vi "check if settings file exists.vi"(8 "error in (no error)":errorcluster, 11 "Autofocus in":refnum<class "Autofocus.lvclass">) -> (0 "error out":errorcluster, 2 "settings file exists?":bool, 3 "Autofocus out":refnum<class "Autofocus.lvclass">)   [LabVIEW 2012, in "Autofocus.lvclass"]
uses:
  Autofocus.lvclass
  <vilib>/Distrio/Murmex/Murmex/Murmex.lvclass
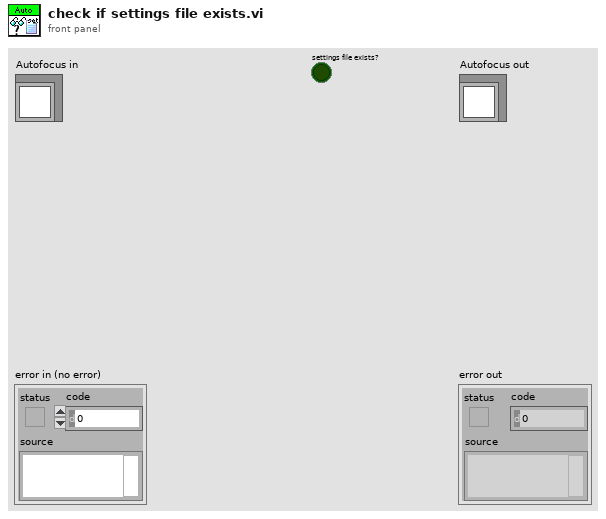
[diagram p1: front panel]
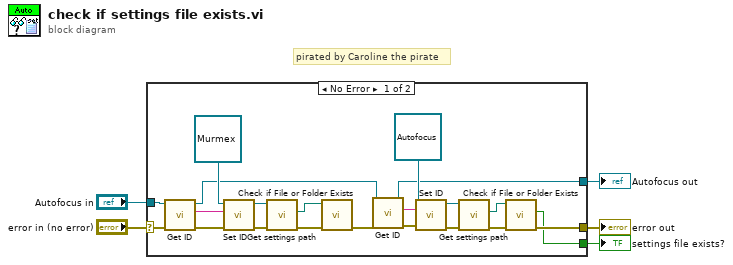
[diagram p0: block diagram]
diagram:
  # "pirated by Caroline the pirate"
  n1 = case shown="No Error" "error in (no error)" {
    selector: "error in (no error)" -> [w19 w28]
    tunnel: [w15 w28] -> w4
    tunnel: [w7 w27] -> w2
    tunnel: "Autofocus in" -> [w25 w27]
    tunnel: [w6 _] -> w1
    frame No Error {
      n2 = call <vilib>:"Get ID.vi"("error in (no error)"=w19, "Murmex in"=w25) -> ("error out"=w23:errorcluster, "component id"=w24:string, "Murmex out"=w8:refnum<class "Autofocus.lvclass">)  [unwired: 7 in]
      n3 = call <vilib>:"Set ID.vi"("error in (no error)"=w23, "id"=w24, "Murmex in"=refnum<class "Murmex.lvclass"> refnum ("GenericComponent.lvclass")) -> ("error out"=w22:errorcluster, "Murmex out"=w21:refnum<class "Murmex.lvclass">)  [unwired: 7 in]
      n4 = call-dynamic "Get settings path.vi"("error in (no error)"=w22, "Murmex in"=w21) -> ("error out"=w20:errorcluster, "settings path"=w18:path)  [unwired: 7 in, 1 out]
      n5 = call <vilib>:"Check if File or Folder Exists.vi"("error in (no error)"=w20, "path"=w18) -> ("error out"=w11:errorcluster)  [unwired: 7 in, 2 out]
      n6 = call <vilib>:"Get ID.vi"("error in (no error)"=w11, "Murmex in"=w8) -> ("error out"=w10:errorcluster, "component id"=w9:string, "Murmex out"=w7:refnum<class "Autofocus.lvclass">)  [unwired: 7 in]
      n7 = call <vilib>:"Set ID.vi"("error in (no error)"=w10, "id"=w9, "Murmex in"=refnum<class "Autofocus.lvclass"> refnum ("Autofocus.lvclass")) -> ("error out"=w16:errorcluster, "Murmex out"=w13:refnum<class "Autofocus.lvclass">)  [unwired: 7 in]
      n8 = call-dynamic "Get settings path.vi"("error in (no error)"=w16, "Autofocus in"=w13) -> ("error out"=w17:errorcluster, "settings path"=w12:path)  [unwired: 7 in, 1 out]
      n9 = call <vilib>:"Check if File or Folder Exists.vi"("error in (no error)"=w17, "path"=w12) -> ("error out"=w15:errorcluster, "file or folder exists?"=w6:bool)  [unwired: 7 in, 1 out]
    }
    frame Error {
    }
  }
  "error out" <- w4
  "Autofocus out" <- w2
  "settings file exists?" <- w1
